vi "Register Window.vi"(8 "error in (no error)":errorcluster caption="错误输入（无错误）", 10 "New Window":T1, 11 "User Interface 输入":refnum<class "User Interface.lvclass">) -> (0 "error out":errorcluster caption="错误输出", 3 "User Interface 输出":refnum<class "User Interface.lvclass">)   [LabVIEW 2018, in "MainInterface.lvlib" / "User Interface.lvclass"]
uses:
  User Interface.lvclass
  Register Window Argument--cluster.ctl
  <vilib>/Delacor/Delacor QMH/Libraries/Message Queue_class/Delacor_lib_QMH_Message Queue.lvclass
  User Interface.lvclass/User Interface.ctl
  MainInterface.lvlib
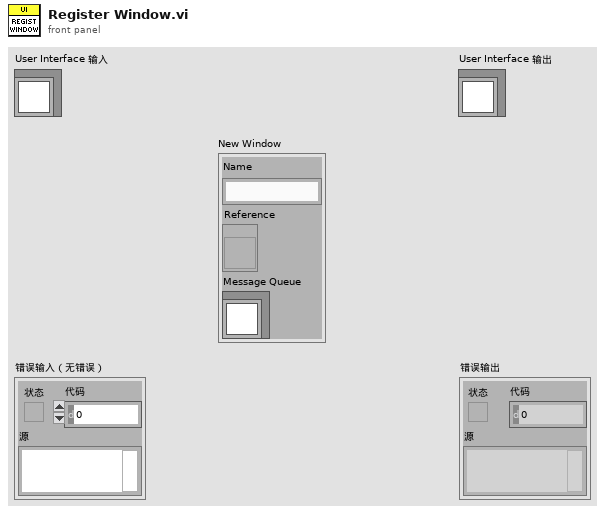
[diagram p1: front panel]
types:
  T1 = typedef "MainInterface.lvlib/Register Window Argument--cluster.ctl" = cluster{"Name":string, "Reference":refnum<vi>, "Message Queue":refnum<class "Delacor_lib_QMH_Message Queue.lvclass">}
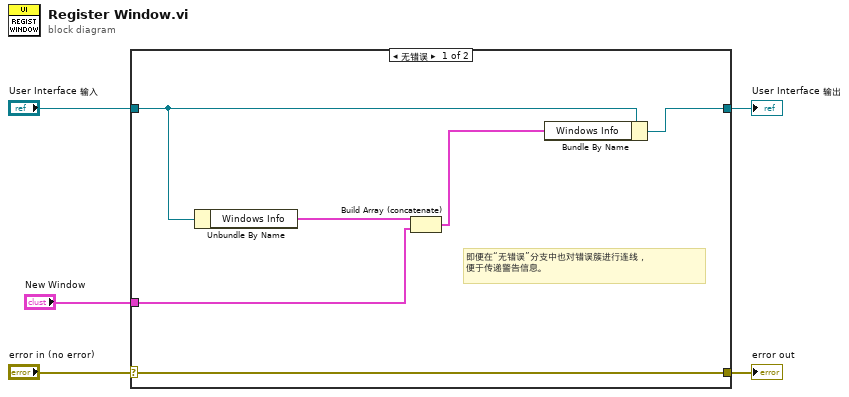
[diagram p0: block diagram]
diagram:
  n1 = case shown="无错误" "error in (no error)" {
    selector: "error in (no error)" -> [w11 w13]
    tunnel: [w11 w13] -> w4
    tunnel: [w8 w12] -> w2
    tunnel: "User Interface 输入" -> [w10 w12]
    tunnel: "New Window" -> [w6 _]
    frame No Error {
      # "即便在“无错误”分支中也对错误簇进行连线，\n便于传递警告信息。"
      n2 = Unbundle By Name(w10) -> ("Windows Info"=w9:T1[])
      n3 = Build Array (concatenate)(w9, w6) -> (w7:T1[])
      n4 = Bundle By Name(cluster=w10, "Windows Info"=w7) -> (w8:refnum<class "User Interface.lvclass">)
    }
    frame Error {
    }
  }
  "error out" <- w4
  "User Interface 输出" <- w2
